vi "parse_wrench.vi"(4 "error in":errorcluster, 7 "msg in":string) -> (0 "error out":errorcluster, 2 "Wrench":T1, 3 "msg out":string)   [LabVIEW 2010]
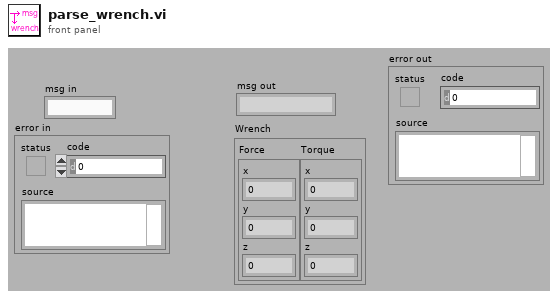
[diagram p1: front panel]
types:
  T1 = cluster{"Force":cluster{"x":dbl, "y":dbl, "z":dbl}, "Torque":cluster{"x":dbl, "y":dbl, "z":dbl}}
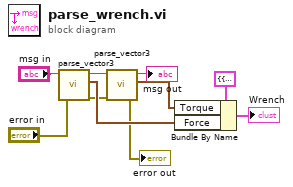
[diagram p0: block diagram]
diagram:
  n1 = call "parse_vector3.vi"("error in"="error in", "msg in"="msg in") -> ("error out"=w3:errorcluster, "Vector3"=w7:cluster{"x":dbl, "y":dbl, "z":dbl}, "msg out"=w10:string)  [unwired: 3 in]
  n2 = call "parse_vector3.vi"("error in"=w3, "msg in"=w10) -> ("error out"=→"error out":errorcluster, "Vector3"=w8:cluster{"x":dbl, "y":dbl, "z":dbl}, "msg out"=→"msg out":string)  [unwired: 3 in]
  n3 = Bundle By Name(cluster=T1 {"Force"={"x"=0.0, "y"=0.0, "z"=0.0}, "Torque"={"x"=0.0, "y"=0.0, "z"=0.0}} ("Wrench"), "Torque"=w8, "Force"=w7) -> (→"Wrench":T1)
